vi "main.vi"() -> ()   [LabVIEW 2023]
doc: "Overview\nThis VI is designed to convert typical response strings from a multimeter into a numerical value formatted in ISO representation. \n\nInputs\nResponse String: A string input representing the multimeter’s response, typically in the form of:\nDC-1.234E-02V\nR4W+5.678E+07OHM\n\nOutputs\nISO Number: The numeric output in ISO format, represented as a double-precision floating-point number.\n\nFunctional Description\n1) String Input: The user inputs a response string from the multimeter into the VI.\n2) Pattern Matching: The VI uses a regular expression to identify and extract the numerical value from the response string.\n3) Conversion to Number: The extracted string is converted to a numerical format.\n4) Output Formatting: The number is formatted in ISO representation and presented as output."
uses:
  <vilib>/Utility/error.llb/Trim Whitespace One-Sided.vi
  <vilib>/regexp/Match Regular Expression.xnode
panel:
  in  "stop":bool
  out "Numeric":dbl format="%#_6p"
  in  "String":string
  # "Determine measured value from result string"
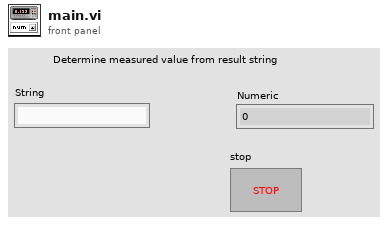
[diagram p1: front panel]
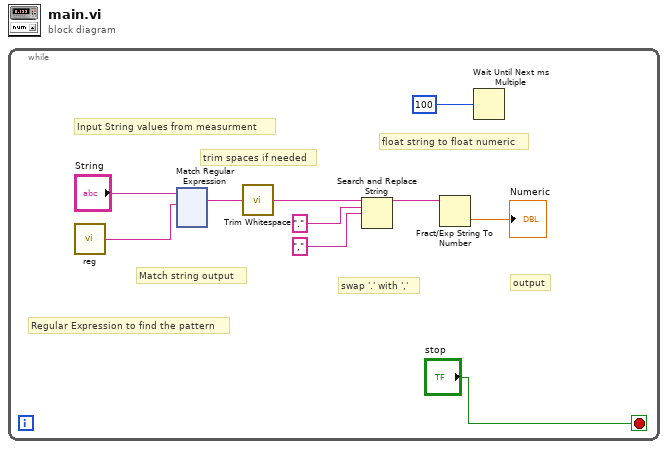
[diagram p0: block diagram]
diagram:
  n1 = while {
    stop <- "stop" stop-if-true
    # "output"
    # "float string to float numeric"
    # "swap '.' with ','"
    # "trim spaces if needed"
    # "Match string output"
    # "Regular Expression to find the pattern"
    # "Input String values from measurment"
    n2 = call "reg.vi"() -> ("String"=w9:string)
    n3 = xnode "Match Regular Expression"("input string"="String", "regular expression"=w9) -> ("whole match"=w8:string)  [unwired: 4 in, 4 out]
    n4 = call <vilib>:"Trim Whitespace.vi"("string"=w8) -> ("trimmed string"=w7:string)  [unwired: 1 in]
    n5 = Search and Replace String(input string=w7, search string=".", replace string=",") -> (result string=w4:string)  [unwired: 5 in, 3 out]
    n6 = Fract/Exp String To Number(string=w4) -> (number=→"Numeric":dbl)  [unwired: 3 in, 1 out]
    n7 = Wait Until Next ms Multiple(millisecond multiple=100) -> ()  [unwired: 1 out]
  }
